vi "configure channel.vi"(5 "user event":T1, 7 "instance id":string, 8 "error in":errorcluster, 9 "line":T2, 10 "engine configuration in":refnum<class "engine configuration.lvclass">, 11 "Scan Engine configuration in":refnum<class "Scan Engine configuration.lvclass">) -> (0 "error out":errorcluster, 2 "engine configuration out":refnum<class "engine configuration.lvclass">, 3 "Scan Engine configuration out":refnum<class "Scan Engine configuration.lvclass">)   [LabVIEW 2013, in "Scan Engine editor node.lvclass"]
uses:
  Scan Engine editor node.lvclass
  <vilib>/NI/TBM Modules/variable/module/configuration/Scan Engine configuration.lvclass
  <vilib>/NI/Module Execution Interface/Engine Configuration/engine configuration.lvclass
  table line.ctl
  <vilib>/NI/Tag Bus Module Framework/channel/TBM channel.lvclass
  <vilib>/CEF_TreeControl/Node/UserEventRef.ctl
  <vilib>/CEF_TreeControl/Controls/EventCluster.ctl
  <vilib>/NI/Tag Bus/tag/tag descriptor.lvclass/tag descriptor.ctl
  <vilib>/NI/Tag Bus/tag/tag descriptor.lvclass
  <vilib>/CEF_TreeControl/NISE_CEF_TreeControl.lvlib
  <vilib>/CEF_TreeControl/Node/NISE_CEF_Node.lvclass
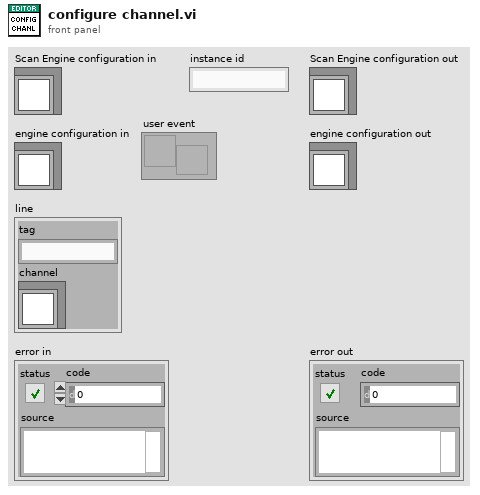
[diagram p1: front panel]
types:
  T1 = typedef "NISE_CEF_Node.lvclass/UserEventRef.ctl" = refnum<user-event>
  T2 = typedef "Scan Engine editor node.lvclass/table line.ctl" = cluster{"tag":string, "channel":refnum<class "TBM channel.lvclass">}
  T3 = typedef "NISE_CEF_TreeControl.lvlib/EventCluster.ctl" = cluster{"command":string, "data":string}
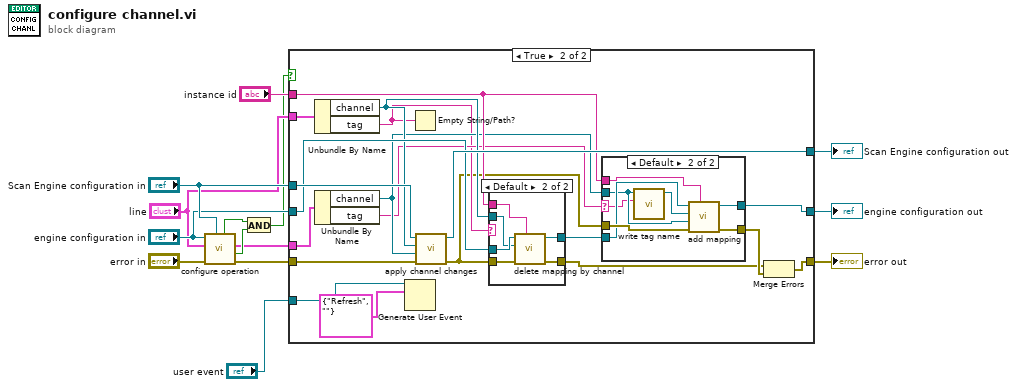
[diagram p0: block diagram]
diagram:
  n1 = call "configure operation.vi"("Scan Engine configuration"="Scan Engine configuration in", "error in"="error in", "line item in"="line", "engine configuration in"="engine configuration in") -> ("error out"=w3:errorcluster, "success"=w8:bool, "line item out"=w4:T2, "changed"=w7:bool)  [unwired: 4 in]
  n2 = And(x=w7, y=w8) -> (x .and. y?=w9:bool)
  n3 = case shown="True" w9 {
    tunnel: [w16 w22] -> w6
    tunnel: [w17 w26] -> w12
    tunnel: "engine configuration in" -> [w17 w31]
    tunnel: w3 -> [w16 w33]
    tunnel: w4 -> [_ w36]
    tunnel: "Scan Engine configuration in" -> [w15 w35]
    tunnel: [w15 w32] -> w5
    tunnel: "instance id" -> [_ w28]
    tunnel: "line" -> [_ w34]
    tunnel: "user event" -> [_ w18]
    frame False {
    }
    frame True {
      n4 = Unbundle By Name(w34) -> ("channel"=w30:refnum<class "TBM channel.lvclass">, "tag"=w23:string)
      n5 = Unbundle By Name(w36) -> ("channel"=w25:refnum<class "TBM channel.lvclass">, "tag"=w24:string)
      n6 = Generate User Event(user event=w18, event data cluster=T3 {"command"="Refresh", "data"=""} ("event data")) -> ()  [unwired: 2 in, 2 out]
      n7 = Empty String/Path?(string/path=w23) -> ()  [unwired: 1 out]
      n8 = call <vilib>:"apply channel changes.vi"("error in"=w33, "new"=w25, "old"=w30, "Scan Engine configuration"=w35) -> ("error out"=w20:errorcluster, "Scan Engine configuration out"=w32:refnum<class "Scan Engine configuration.lvclass">)  [unwired: 6 in]
      n9 = case shown="Default" w23 {
        tunnel: w20 -> [w37 w44]
        tunnel: w31 -> [w38 w43]
        tunnel: w30 -> [_ w42]
        tunnel: [w37 w41] -> w21
        tunnel: w28 -> [_ w40]
        tunnel: [w38 w39] -> w27
        frame "" {
        }
        frame Default {
          n10 = call <vilib>:"delete mapping by channel.vi"("owner ID"=w40, "error in"=w44, "channel"=w42, "engine configuration in"=w43) -> ("error out"=w41:errorcluster, "engine configuration out"=w39:refnum<class "engine configuration.lvclass">)  [unwired: 6 in]
        }
      }
      n11 = case shown="Default" w24 {
        selector: w24 -> [_ w47]
        tunnel: w20 -> [w45 w54]
        tunnel: [w45 w53] -> w29
        tunnel: w28 -> [_ w52]
        tunnel: w27 -> [w46 w51]
        tunnel: [w46 w50] -> w26
        tunnel: w25 -> [_ w48]
        frame "" {
        }
        frame Default {
          n12 = call <vilib>:"write tag name.vi"("name"=w47, "system tag in"=w48) -> ("system tag out"=w49:refnum<class "TBM channel.lvclass">)  [unwired: 8 in, 1 out]
          n13 = call <vilib>:"add mapping.vi"("owner ID"=w52, "error in"=w54, "channel"=w48, "tag descriptor"=w49, "engine configuration"=w51) -> ("error out"=w53:errorcluster, "engine configuration out"=w50:refnum<class "engine configuration.lvclass">)  [unwired: 5 in]
        }
      }
      n14 = Merge Errors(w21, w29) -> (w22:errorcluster)
    }
  }
  "engine configuration out" <- w12
  "error out" <- w6
  "Scan Engine configuration out" <- w5
